vi "RuO2 1k5.vi"(1 "temperature \n(OR resistance)":dbl) -> (0 "resistance \n(OR temperature)":dbl)   [LabVIEW 2013]
panel:
  # "This tool convert data for a 1.5K thermometer (RuO2). Edit \nconstants in the block diagram to modify calibration."
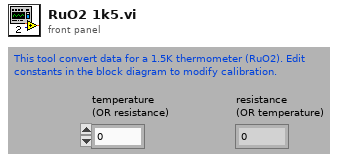
[diagram p1: front panel]
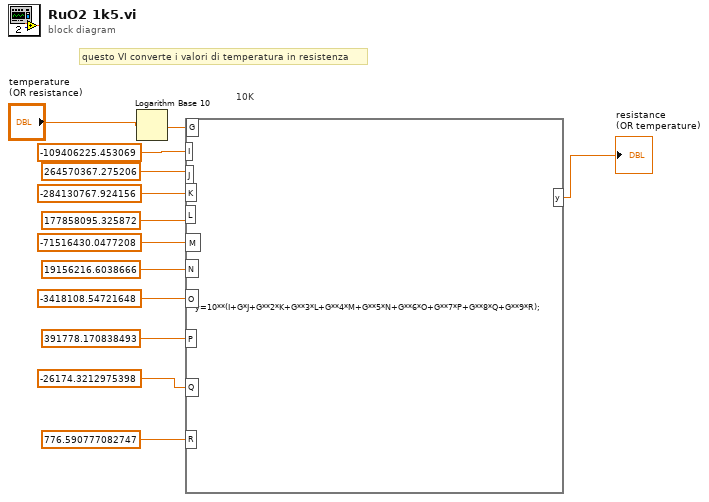
[diagram p0: block diagram]
diagram:
  # "10K"
  # "questo VI converte i valori di temperatura in resistenza"
  n1 = Logarithm Base 10(1:"temperature \n(OR resistance)") -> (0:w13:dbl)
  n2 = formula code="y=10**(I+G*J+G**2*K+G**3*L+G**4*M+G**5*N+G**6*O+G**7*P+G**8*Q+G**9*R);"("G"=w13, "I"=-109406225.453069 ("input variable"), "L"=177858095.325872 ("input variable"), "M"=-71516430.0477208 ("input variable"), "O"=-3418108.54721648 ("input variable"), "Q"=-26174.3212975398 ("input variable"), "R"=776.590777082747 ("input variable"), "P"=391778.170838493 ("input variable"), "N"=19156216.6038666 ("input variable"), "J"=264570367.275206 ("input variable"), "K"=-284130767.924156 ("input variable")) -> ("y"=→"resistance \n(OR temperature)":dbl)
